vi "StimProfilePathBuilder.vi"(8 "Stim profile path":string, 9 "Stim profile":string, 10 "Working Directory":string) -> (1 "VS Log file":string, 2 "Stim Parameters":string[](array[string]))   [LabVIEW 2010]
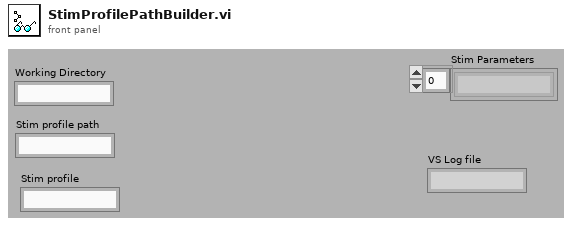
[diagram p1: front panel]
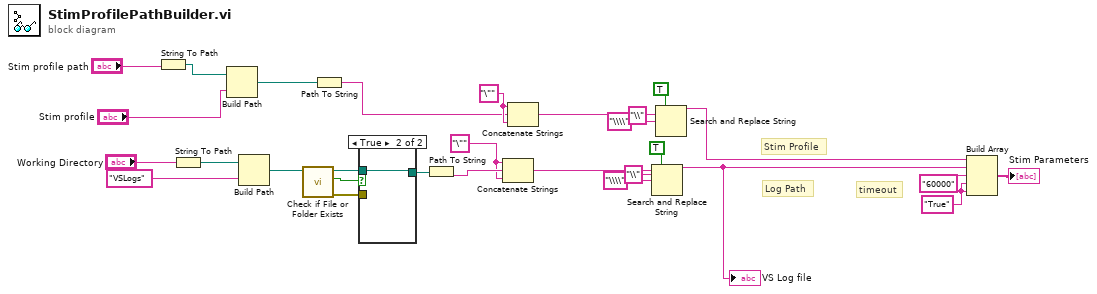
[diagram p0: block diagram]
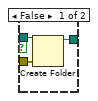
[diagram p2: hidden frame]
diagram:
  w15 = "\"" ("string")
  w18 = "True" ("element")
  w24 = "\"" ("string")
  # "Stim Profile"
  # "timeout"
  # "Log Path"
  n1 = String To Path(string="Stim profile path") -> (path=w4:path)
  n2 = String To Path(string="Working Directory") -> (path=w6:path)
  n3 = Build Path(base path=w4, name or relative path="Stim profile") -> (appended path=w2:path)
  n4 = Build Path(base path=w6, name or relative path="VSLogs") -> (appended path=w9:path)
  n5 = call <vilib>:"Check if File or Folder Exists.vi"("path"=w9) -> ("error out"=w14:errorcluster, "file or folder exists?"=w11:bool, "dup path"=w13:path)  [unwired: 8 in]
  n6 = Path To String(path=w2) -> (string=w1:string)
  n7 = case shown="True" w11 {
    tunnel: w14 -> [w32 _]
    tunnel: w13 -> [w31 w33]
    tunnel: [w30 w33] -> w12
    frame False {
      n8 = Create Folder(path (use dialog)=w31, error in=w32) -> (created path=w30:path)  [unwired: 1 in, 2 out]
    }
    frame True {
    }
  }
  n9 = Path To String(path=w12) -> (string=w25:string)
  n10 = Concatenate Strings(w24, w25, w24) -> (w20:string)
  n11 = Concatenate Strings(w15, w1, w15) -> (w29:string)
  n12 = Search and Replace String(replace all?=TRUE ("replace all? (F)"), input string=w20, search string="\\", replace string="\\\\" ("replace string (\"\")")) -> (result string=w7:string)  [unwired: 4 in, 3 out]
  "VS Log file" <- w7
  n13 = Search and Replace String(replace all?=TRUE ("replace all? (F)"), input string=w29, search string="\\", replace string="\\\\" ("replace string (\"\")")) -> (result string=w16:string)  [unwired: 4 in, 3 out]
  n14 = Build Array(w16, w7, "60000" ("element"), w18, w18) -> (→"Stim Parameters":string[])
